vi "Close Refs.vi"(8 "RT Data In":refnum<class "DCM-NIVS-RT.lvclass">, 11 "error in":errorcluster) -> (3 "error out":errorcluster)   [LabVIEW 2016, in "DCM Engine.lvlib" / "DCM-NIVS-RT.lvclass"]
uses:
  DCM-NIVS-RT.lvclass
  DCM-NIVS-RT.lvclass/DCM-NIVS-RT.ctl
  Built/DCM Classes Packed/Pharlap/C/DCM-Classes.lvlibp/DCM/Rev0/RT/DCM - RT.lvclass
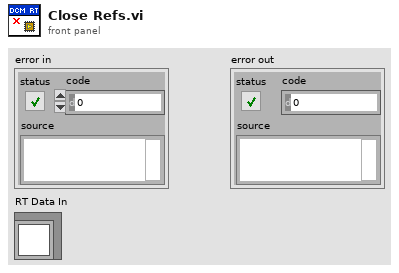
[diagram p1: front panel]
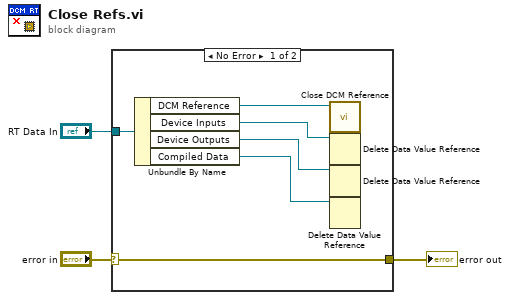
[diagram p0: block diagram]
diagram:
  n1 = case shown="No Error" "error in" {
    selector: "error in" -> [w9 w10]
    tunnel: [w9 w10] -> w2
    tunnel: "RT Data In" -> [w5 _]
    frame No Error {
      n2 = Unbundle By Name(w5) -> ("DCM Reference"=w4:refnum<class "DCM - RT.lvclass">, "Device Inputs"=w6:refnum<data-value>, "Device Outputs"=w7:refnum<data-value>, "Compiled Data"=w8:refnum<data-value>)
      n3 = call "Close DCM Reference.vi"("DCM - RT in"=w4) -> ()  [unwired: 11 in]
      n4 = Delete Data Value Reference(data value reference=w6) -> ()  [unwired: 1 in, 2 out]
      n5 = Delete Data Value Reference(data value reference=w7) -> ()  [unwired: 1 in, 2 out]
      n6 = Delete Data Value Reference(data value reference=w8) -> ()  [unwired: 1 in, 2 out]
    }
    frame Error {
    }
  }
  "error out" <- w2
